vi "Define Criteria.vi"(10 "Criteria":T1, 11 "UniquenessCriteria in":refnum<class "UniquenessCriteria.lvclass">) -> (3 "UniquenessCriteria out":refnum<class "UniquenessCriteria.lvclass">)   [LabVIEW 2014, in "UniquenessCriteria.lvclass"]
uses:
  UniquenessCriteria.lvclass
  Criteria.ctl
  UniquenessCriteria.lvclass/UniquenessCriteria.ctl
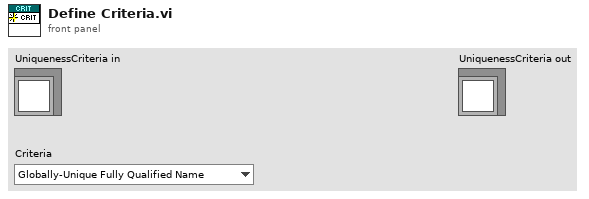
[diagram p1: front panel]
types:
  T1 = typedef "UniquenessCriteria.lvclass/Criteria.ctl" = enum16{"Globally-Unique Fully Qualified Name", "Globally-Unique Name"}
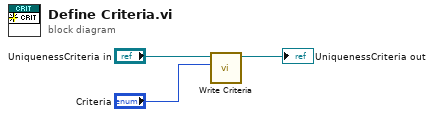
[diagram p0: block diagram]
diagram:
  n1 = call "Write Criteria.vi"("Criteria"="Criteria", "UniquenessCriteria in"="UniquenessCriteria in") -> ("UniquenessCriteria out"=→"UniquenessCriteria out":refnum<class "UniquenessCriteria.lvclass">)  [unwired: 9 in]
